vi "Pre Launch Init.vi"(11 "Grayscale in":refnum<class "Grayscale.lvclass">) -> (0 "error out":errorcluster, 3 "Grayscale out":refnum<class "Grayscale.lvclass">)   [LabVIEW 2016, in "Tests.lvlib" / "Grayscale.lvclass"]
doc: "This VI creates User events for the actor to receive messages from other actors."
uses:
  Grayscale.lvclass
  <vilib>/ActorFramework/Message Enqueuer/Message Enqueuer.lvclass
  <vilib>/vision/Image Controls.llb/IMAQ Image.ctl
  Grayscale.lvclass/Grayscale.ctl
  Tests.lvclass
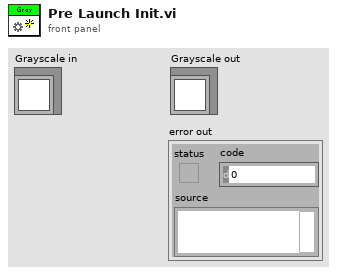
[diagram p1: front panel]
types:
  T1 = typedef "IMAQ Image.ctl" = refnum<image>
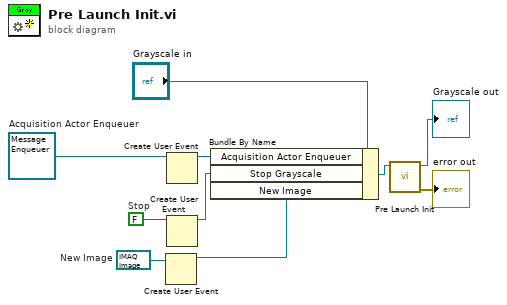
[diagram p0: block diagram]
diagram:
  w2 = T1 refnum  # New Image
  w8 = FALSE  # Stop
  w5 = refnum<class "Message Enqueuer.lvclass"> refnum  # Acquisition Actor Enqueuer
  n1 = Create User Event(user event datatype=w2) -> (user event=w1:refnum<user-event>)  [unwired: 1 in, 1 out]
  n2 = Create User Event(user event datatype=w5) -> (user event=w7:refnum<user-event>)  [unwired: 1 in, 1 out]
  n3 = Create User Event(user event datatype=w8) -> (user event=w6:refnum<user-event>)  [unwired: 1 in, 1 out]
  n4 = Bundle By Name(cluster="Grayscale in", "Acquisition Actor Enqueuer"=w7, "Stop Grayscale"=w6, "New Image"=w1) -> (w3:refnum<class "Grayscale.lvclass">)
  n5 = call-parent "Pre Launch Init.vi"("Actor in"=w3) -> ("error out"=→"error out":errorcluster, "Actor out"=→"Grayscale out":refnum<class "Grayscale.lvclass">)  [unwired: 9 in]
